vi "AIT 664 - Extract Channel Information.vi"(0 "Channel Refs":T1[](array[typedef]) format="%.0x", 5 "Parent Guid":string, 11 "error in (no error)":errorcluster) -> (4 "Parameters out":T2[](array[typedef]), 15 "error out":errorcluster)   [LabVIEW 2013, in "AIT 664 Custom Device.lvlib"]
doc: "Given the channels for a system exract the parameter information"
uses:
  Controls/664 -Param.ctl
  <vilib>/NI Veristand/Custom Device API/Custom Device Item Ref.ctl
  <vilib>/NI Veristand/Custom Device API/Get Item Property (I32).vi
  <vilib>/NI Veristand/Custom Device API/Get Item Property (Double).vi
  <vilib>/NI Veristand/Custom Device API/Get Item Property (Boolean).vi
  AIT 664 Custom Device.lvlib
  <vilib>/NI Veristand/Custom Device API/Custom Device API.lvlib
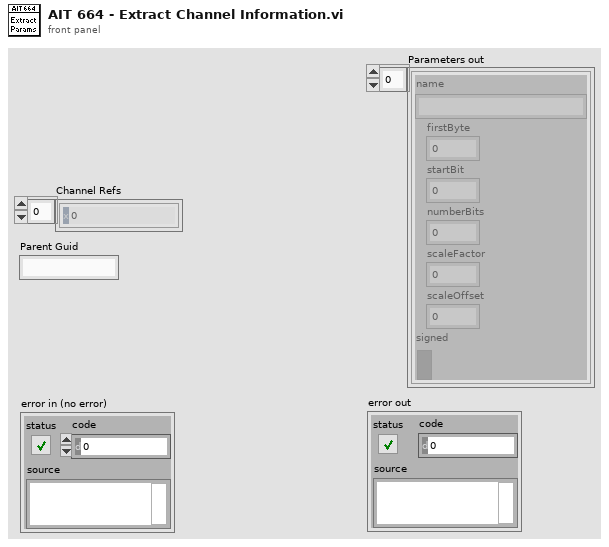
[diagram p1: front panel]
types:
  T1 = typedef "Custom Device API.lvlib/Custom Device Item Ref.ctl" = u64
  T2 = typedef "AIT 664 Custom Device.lvlib/664 -Param.ctl" = cluster{"name":string, "firstByte":i32, "startBit":i32, "numberBits":i32, "scaleFactor":dbl, "scaleOffset":dbl, "signed":bool}
  T3 = typedef "Custom Device API.lvlib/Custom Device Item Info.ctl" = cluster{"Name":string, "Is Channel":bool, "GUID":string, "Is Waveform":bool}
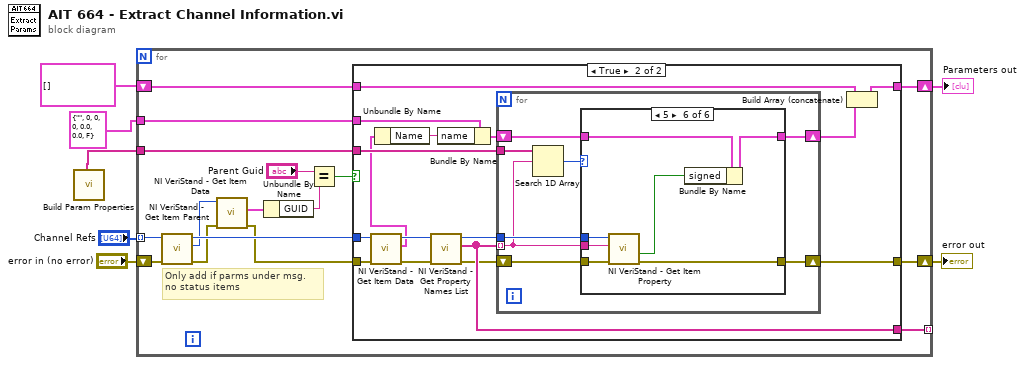
[diagram p0: block diagram]
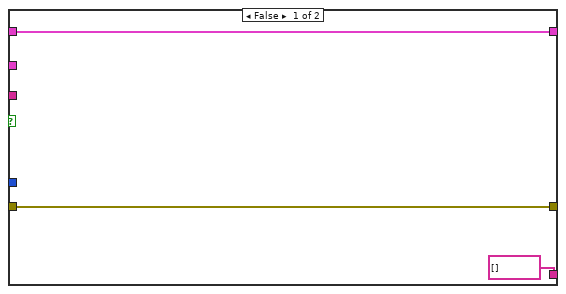
[diagram p2: hidden frame]
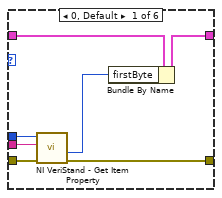
[diagram p3: hidden frame]
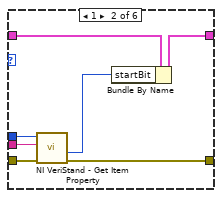
[diagram p4: hidden frame]
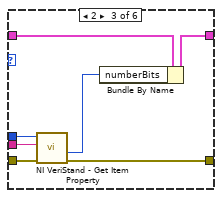
[diagram p5: hidden frame]
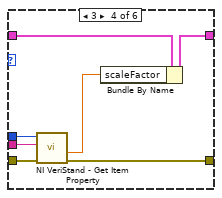
[diagram p6: hidden frame]
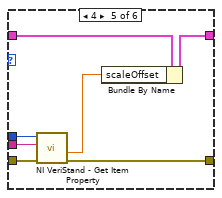
[diagram p7: hidden frame]
diagram:
  n1 = call "Build Param Properties.vi"() -> ("Prop Names"=w6:string[])  [unwired: 11 in, 8 out]
  n2 = for {
    tunnel: "Channel Refs" -> [w16] mode=indexing
    tunnel: w6 -> [w23]
    tunnel: [w21] -> _ mode=indexing
    tunnel: T2 {"name"="", "firstByte"=0, "startBit"=0, "numberBits"=0, "scaleFactor"=0.0, "scaleOffset"=0.0, "signed"=FALSE} ("1553 Parameter") -> [w22]
    shift-right: [w19] -> w7
    shift-left: T2[] [] -> [w20]
    shift-right: [w18] -> w1
    shift-left: "error in (no error)" -> [w17]
    # "Only add if parms under msg.\nno status items"
    n3 = call <vilib>:"NI VeriStand - Get Item Parent.vi"("error in (no error)"=w17, "Item Ref in"=w16) -> ("error out"=w14:errorcluster, "Parent Ref"=w12:T1, "Item Ref out"=w15:T1)  [unwired: 6 in, 1 out]
    n4 = call <vilib>:"NI VeriStand - Get Item Data.vi"("error in (no error)"=w14, "Item Ref in"=w12) -> ("error out"=w13:errorcluster, "Item Info"=w11:T3)  [unwired: 6 in, 2 out]
    n5 = Unbundle By Name(w11) -> ("GUID"=w9:string)
    n6 = Equal?(x="Parent Guid", y=w9) -> (x = y?=w10:bool)
    n7 = case shown="True" w10 {
      tunnel: w23 -> [_ w42]
      tunnel: w22 -> [_ w41]
      tunnel: [string[] [] ("Property Names") w40] -> w21
      tunnel: w20 -> [w26 w39]
      tunnel: [w26 w38] -> w19
      tunnel: [w25 w29] -> w18
      tunnel: w15 -> [_ w28]
      tunnel: w13 -> [w25 w27]
      frame False {
      }
      frame True {
        n8 = call <vilib>:"NI VeriStand - Get Item Data.vi"("error in (no error)"=w27, "Item Ref in"=w28) -> ("error out"=w35:errorcluster, "Item Info"=w31:T3, "Item Ref out"=w34:T1)  [unwired: 6 in, 1 out]
        n9 = Unbundle By Name(w31) -> ("Name"=w32:string)
        n10 = call <vilib>:"NI VeriStand - Get Property Names List.vi"("error in (no error)"=w35, "Item Ref in"=w34) -> ("error out"=w37:errorcluster, "Property Names"=w40:string[], "Item Ref out"=w36:T1)  [unwired: 7 in]
        n11 = Bundle By Name(cluster=w41, "name"=w32) -> (w33:T2)
        n12 = for {
          tunnel: w40 -> [w45] mode=indexing
          tunnel: w42 -> [w50]
          shift-right: [w44] -> w30
          shift-left: w33 -> [w48]
          tunnel: w36 -> [w46]
          shift-right: [w43] -> w29
          shift-left: w37 -> [w47]
          n13 = Search 1D Array(1D array=w50, element=w45) -> (index of element=w49:i32)  [unwired: 1 in]
          n14 = case shown="5" w49 {
            tunnel: w48 -> [w57 w64 w71 w78 w85 w92]
            tunnel: w47 -> [w56 w63 w70 w77 w84 w91]
            tunnel: w46 -> [w55 w62 w69 w76 w83 w90]
            tunnel: w45 -> [w54 w61 w68 w75 w82 w89]
            tunnel: [w52 w59 w66 w73 w80 w87] -> w44
            tunnel: [w51 w58 w65 w72 w79 w86] -> w43
            frame 0, Default {
              n15 = call-poly <vilib>:"NI VeriStand - Get Item Property.vi"("error in (no error)"=w56, "Property Name"=w54, "Item Ref in"=w55) -> ("error out"=w51:errorcluster, "Value"=w53:i32)  [unwired: 5 in, 2 out]
              n16 = Bundle By Name(cluster=w57, "firstByte"=w53) -> (w52:T2)
            }
            frame 1 {
              n17 = call-poly <vilib>:"NI VeriStand - Get Item Property.vi"("error in (no error)"=w63, "Property Name"=w61, "Item Ref in"=w62) -> ("error out"=w58:errorcluster, "Value"=w60:i32)  [unwired: 5 in, 2 out]
              n18 = Bundle By Name(cluster=w64, "startBit"=w60) -> (w59:T2)
            }
            frame 2 {
              n19 = call-poly <vilib>:"NI VeriStand - Get Item Property.vi"("error in (no error)"=w70, "Property Name"=w68, "Item Ref in"=w69) -> ("error out"=w65:errorcluster, "Value"=w67:i32)  [unwired: 5 in, 2 out]
              n20 = Bundle By Name(cluster=w71, "numberBits"=w67) -> (w66:T2)
            }
            frame 3 {
              n21 = call-poly <vilib>:"NI VeriStand - Get Item Property.vi"("error in (no error)"=w77, "Property Name"=w75, "Item Ref in"=w76) -> ("error out"=w72:errorcluster, "Value"=w74:dbl)  [unwired: 5 in, 2 out]
              n22 = Bundle By Name(cluster=w78, "scaleFactor"=w74) -> (w73:T2)
            }
            frame 4 {
              n23 = call-poly <vilib>:"NI VeriStand - Get Item Property.vi"("error in (no error)"=w84, "Property Name"=w82, "Item Ref in"=w83) -> ("error out"=w79:errorcluster, "Value"=w81:dbl)  [unwired: 5 in, 2 out]
              n24 = Bundle By Name(cluster=w85, "scaleOffset"=w81) -> (w80:T2)
            }
            frame 5 {
              n25 = call-poly <vilib>:"NI VeriStand - Get Item Property.vi"("error in (no error)"=w91, "Property Name"=w89, "Item Ref in"=w90) -> ("error out"=w86:errorcluster, "Value"=w88:bool)  [unwired: 5 in, 2 out]
              n26 = Bundle By Name(cluster=w92, "signed"=w88) -> (w87:T2)
            }
          }
        }
        n27 = Build Array (concatenate)(w39, w30) -> (w38:T2[])
      }
    }
  }
  "Parameters out" <- w7
  "error out" <- w1
